vi "Untitled 8 (SubVI).vi"(9 "Cluster 2":T2, 10 "spec cluster in":cluster{"xi used":dbl[], "yi":dbl[]}, 11 "specInfo":T1 {"Charge [pC]" format="%0.4f"}) -> (1 "cHARGE":dbl[][](array[numeric]), 2 "online":dbl[][](array[numeric]), 3 "spec cluster out":cluster{dbl[], dbl[]}, 4 "post":dbl[][](array[numeric]))   [LabVIEW 2011, in "MagAnalysis_Online.lvclass"]
uses:
  MagAnalysis_Online.lvclass
  fileCluster_TypDef.ctl
  specInfo_TypDef.ctl
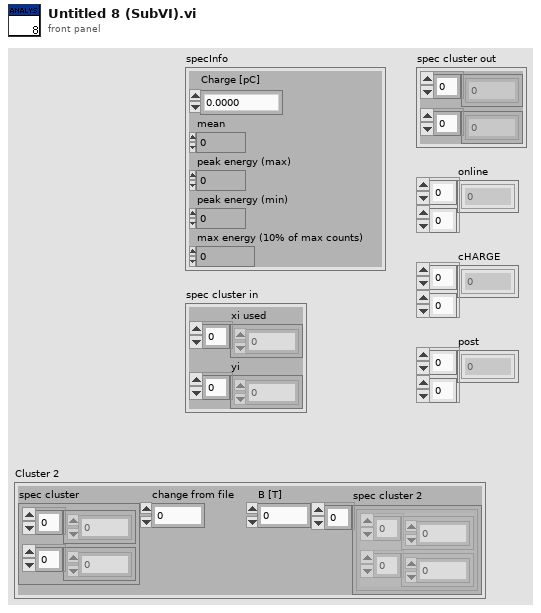
[diagram p1: front panel]
types:
  T1 = typedef "specInfo_TypDef.ctl" = cluster{"Charge [pC]":dbl, "mean":dbl, "peak energy (max)":dbl, "peak energy (min)":dbl, "max energy (10% of max counts)":dbl}
  T2 = typedef "fileCluster_TypDef.ctl" = cluster{"spec cluster":cluster{dbl[], dbl[]}, "change from file":dbl, "B [T]":dbl, "spec cluster 2":cluster{dbl[], dbl[]}[]}
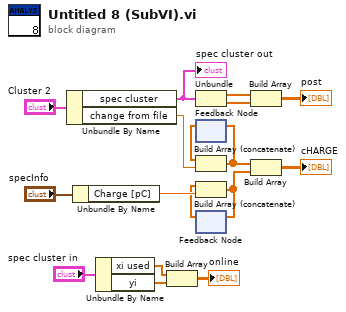
[diagram p0: block diagram]
diagram:
  n1 = Unbundle By Name("Cluster 2") -> ("spec cluster"=w14:cluster{dbl[], dbl[]}, "change from file"=w13:dbl)
  "spec cluster out" <- w14
  n2 = Unbundle By Name("specInfo") -> ("Charge [pC]"=w4:dbl)
  n3 = Unbundle By Name("spec cluster in") -> ("xi used"=w9:dbl[], "yi"=w10:dbl[])
  n4 = Build Array(w9, w10) -> (→"online":dbl[][])
  n5 = Unbundle(w14) -> (w15:dbl[], w16:dbl[])
  n6 = feedback #1() -> (w1:dbl[])  [unwired: 1 in]
  n7 = Build Array (concatenate)(w1, w13) -> (w5:dbl[])
  n8 = feedback-in #1(w5) -> ()
  n9 = feedback #2() -> (w2:dbl[])  [unwired: 1 in]
  n10 = Build Array (concatenate)(w2, w4) -> (w6:dbl[])
  n11 = feedback-in #2(w6) -> ()
  n12 = Build Array(w15, w16) -> (→"post":dbl[][])
  n13 = Build Array(w5, w6) -> (→"cHARGE":dbl[][])
